vi "mod_GenerateFilterCoefficients.vi"(9 "interpolation factor":i32=128, 10 "# of zero crossings":i32=16) -> (0 "full array size":i32, 1 "Differences (scaled)":dbl[](graph), 2 "Filter Coefficients (scaled)":dbl[](graph), 3 "Filter Coefficients (unscaled)":dbl[](graph))   [LabVIEW 2020, in "niAMT.lvlib"]
uses:
  <vilib>/addons/Modulation/niAMT.lvlib
  <vilib>/Analysis/4window.llb/windowTd.ctl
  <vilib>/Analysis/NI_AALBase.lvlib
  <vilib>/Analysis/NI_AALPro.lvlib
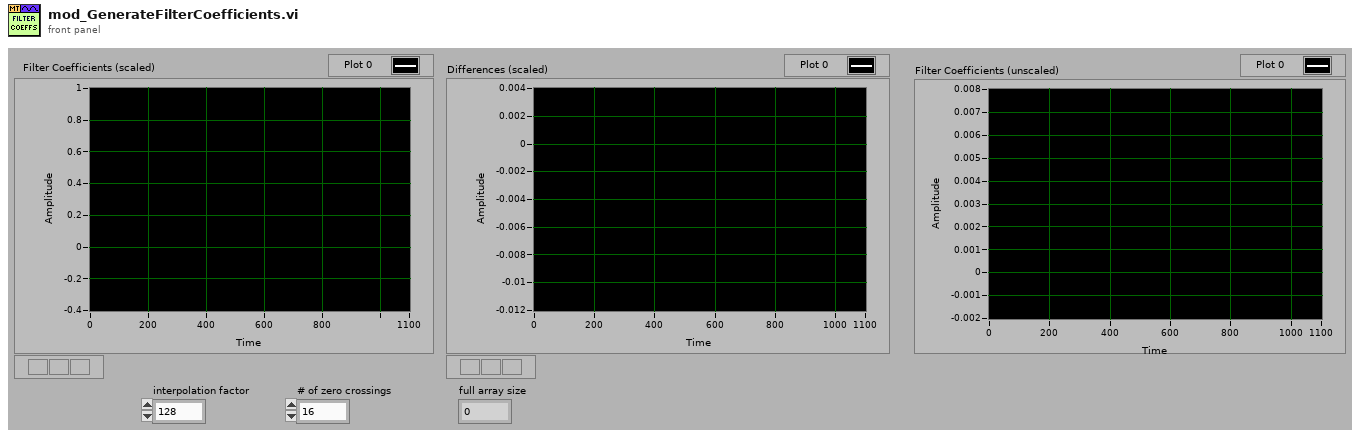
[diagram p1: front panel]
types:
  T1 = typedef "NI_AALPro.lvlib/windowTd.ctl" = u32
  T2 = enum32{"Lowpass", "Highpass", "Bandpass", "Bandstop"}
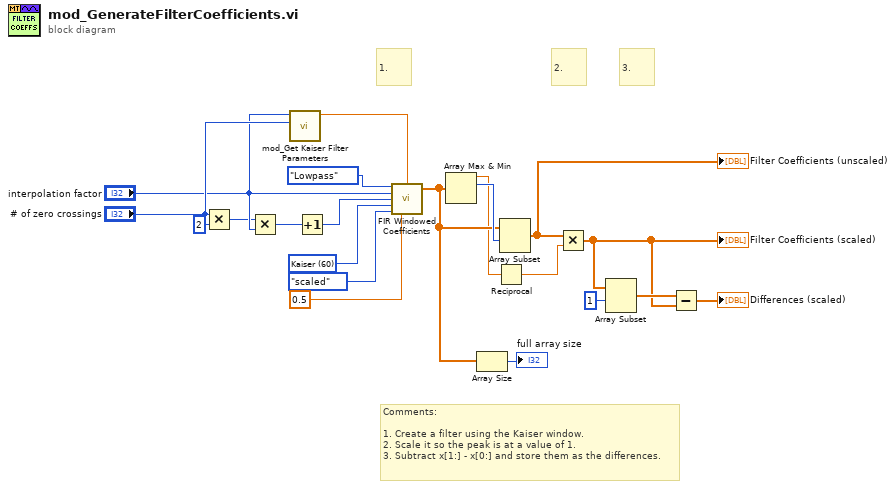
[diagram p0: block diagram]
diagram:
  w14 = T1 60 items=["Rectangle"=0, "Hanning"=1, "Hamming"=2, "Blackman-Harris"=3, "Exact Blackman"=4, "Blackman"=5, "Flat Top"=6, "4 Term B-Harris "=7, "7 Term B-Harris"=8, "Low Sidelobe"=9, "Blackman Nuttall"=11, "Triangle"=30, "Bartlett-Hanning"=31, "Bohman"=32, "Parzen"=33, "Welch"=34, "Kaiser"=60, "Dolph-Chebyshev"=61, "Gaussian"=62] ("window")
  # "Comments:\n\n1. Create a filter using the Kaiser window.\n2. Scale it so the peak is at a value of 1.\n3. Subtract x[1:] - x[0:] and store them as the differences."
  # "3."
  # "2."
  # "1."
  n1 = Multiply(x="# of zero crossings", y=2) -> (x*y=w6:i32)
  n2 = Multiply(x=w6, y="interpolation factor") -> (x*y=w7:i32)
  n3 = call <vilib>:"mod_Get Kaiser Filter Parameters.vi"("len"="# of zero crossings", "I"="interpolation factor") -> ("beta"=w3:dbl)  [unwired: 2 in, 7 out]
  n4 = Increment(x=w7) -> (x+1=w4:i32)
  n5 = call <vilib>:"FIR Windowed Coefficients.vi"("filter type"=T2."Lowpass", "window parameter"=w3, "sampling freq: fs"="interpolation factor", "taps"=w4, "window"=w14, "option"=enum32{"not scaled", "scaled"}."scaled", "low cutoff freq: fl"=0.5) -> ("FIR Windowed Coefficients"=w9:dbl[])  [unwired: 1 in, 7 out]
  n6 = Array Max & Min(array=w9) -> (max value=w2:dbl, max index (indices)=w11:i32)  [unwired: 2 out]
  n7 = Array Size(array=w9) -> (size(s)=→"full array size":i32)
  n8 = Reciprocal(x=w2) -> (1/x=w1:dbl)
  n9 = Array Subset(array=w9, index=w11) -> (w21:dbl[])  [unwired: 1 in]
  "Filter Coefficients (unscaled)" <- w21
  n10 = Multiply(x=w21, y=w1) -> (x*y=w19:dbl[])
  "Filter Coefficients (scaled)" <- w19
  n11 = Array Subset(array=w19, index=1) -> (w20:dbl[])  [unwired: 1 in]
  n12 = Subtract(x=w20, y=w19) -> (x-y=→"Differences (scaled)":dbl[])
